vi "read.vi"(8 "error in (no error)":errorcluster, 9 "bytes to read":i32, 11 "file descriptor in":i32) -> (0 "error out":errorcluster, 1 "bytes read":i32, 2 "data":string, 3 "file descriptor out":i32)   [LabVIEW 2013, in "Pipes.lvlib"]
uses:
  Pipes.lvlib
  Controls/functions.ctl
  <vilib>/NI/NI Linux RT Errno/Linux Errno.lvlib
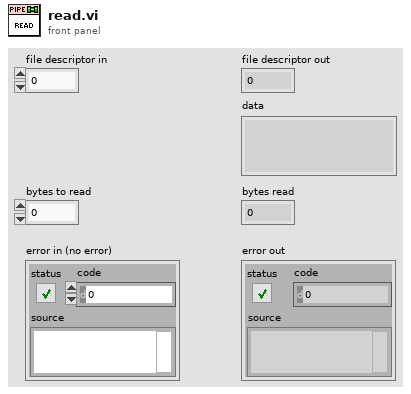
[diagram p1: front panel]
types:
  T1 = typedef "Pipes.lvlib/functions.ctl" = enum16{"unspecified", "mkfifo", "open", "read", "write", "close", "unlink"}
  T2 = typedef "Linux Errno.lvlib/errno.ctl" = enum16{"NO ERROR", "EPERM", "ENOENT", "ESRCH", "EINTR", "EIO", "ENXIO", "E2BIG", "ENOEXEC", "EBADF", "ECHILD", "EAGAIN", "ENOMEM", "EACCES", "EFAULT", "ENOTBLK", "EBUSY", "EEXIST", "EXDEV", "ENODEV", "ENOTDIR", "EISDIR", "EINVAL", "ENFILE", "EMFILE", "ENOTTY", "ETXTBSY", "EFBIG", "ENOSPC", "ESPIPE", "EROFS", "EMLINK", "EPIPE", "EDOM", "ERANGE", "EDADLK", "ENAMETOOLONG", "ENOLCK", "ENOSYS", "ENOTEMPTY", "ELOOP", "EWOULDBLOCK", "ENOMSG", "EIDRM", "ECHRNG", "EL2NSYNC", "EL3HLT", "EL3RST", "ELNRNG", "EUNATCH", "ENOCSI", "EL2HLT", "EBADE", "EBADR", "EXFULL", "ENOANO", "EBADRQC", "EBADSLT", "EDEADLOCK", "EBFONT", "ENOSTR", "ENODATA", "ETIME", "ENOSR", "ENONET", "ENOPKG", "EREMOTE", "ENOLINK", "EADV", "ESRMNT", "ECOMM", "EPROTO", "EMULTIHOP", "EDOTDOT", "EBADMSG", "EOVERFLOW", "ENOTUNIQ", "EBADFD", "EREMCHG", "ELIBACC", "ELIBBAD", "ELIBSCN", "ELIBMAX", "ELIBEXEC", "ELISEQ", "ERESTART", "ESTRPIPE", "EUSERS", "ENOTSOCK", "EDESTADDRREQ", "EMSGSIZE", "EPROTOTYPE", "ENOPROTOOPT", "EPROTONOSUPPORT", "ESOCKTNOSUPPORT", "EOPNOTSUPP", "EPFNOSUPPORT", "EAFNOSUPPORT", "EADDRINUSE", "EADDRNOTAVAIL", "ENETDOWN", "ENETUNREACH", "ENETRESET", "ECONNABORTED", "ECONNRESET", "ENOBUFS", "EISCONN", "ENOTCONN", "ESHUTDOWN", "ETOOMANYREFS", "ETIMEDOUT", "ECONNREFUSED", "EHOSTDOWN", "EHOSTUNREACH", "EALREADY", "EINPROGRESS", "ESTALE", "EUCLEAN", "ENOTNAM", "ENAVAIL", "EISNAM", "EREMOTEIO", "EDQUOT", "ENOMEDIUM", "EMEDIUMTYPE", "ECANCELED", "ENOKEY", "EKEYEXPIRED", "EKEYREVOKED", "EKEYREJECTED", "EOWNERDEAD", "ENOTRECOVERABLE", "ERFKILL", "EHWPOISON", "UNDEFINED"}
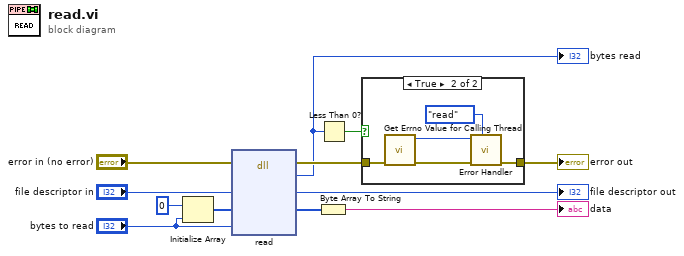
[diagram p0: block diagram]
diagram:
  n1 = Initialize Array(u8 0 ("element"), "bytes to read") -> (w7:u8[])
  n2 = dll-call lib="LabVIEW" fn="read"(error in="error in (no error)", "fd"="file descriptor in", "buf"=w7, "count"="bytes to read") -> (error out=w4:errorcluster, "return"=w1:i32, "fd"=→"file descriptor out":i32, "buf"=w6:u8[])  [unwired: 3 in, 1 out]
  "bytes read" <- w1
  n3 = Byte Array To String(unsigned byte array=w6) -> (string=→"data":string)
  n4 = Less Than 0?(x=w1) -> (x < 0?=w3:bool)
  n5 = case shown="True" w3 {
    tunnel: w4 -> [w13 w18]
    tunnel: [w13 w16] -> w2
    frame False {
    }
    frame True {
      n6 = call <vilib>:"Get Errno Value for Calling Thread.vi"("error in (no error)"=w18) -> ("error out"=w14:errorcluster, "errno"=w15:T2)  [unwired: 9 in]
      n7 = call "Error Handler.vi"("function (unspecified)"=functions."read", "error in (no error)"=w14, "errno"=w15) -> ("error out"=w16:errorcluster)  [unwired: 8 in]
    }
  }
  "error out" <- w2
